vi "FTDI SPI SYS Set.vi"(4 "nCS":u8 max=4 step=1, 5 "ClockRate":u32=50000, 6 "Set Out (0-7)":bool[](array[boolean]), 8 "Use Extra":bool, 10 "Addr":T1 items=["Addr-0", "Addr-1", "Addr-2", "Addr-3", "Addr-4", "Addr-5", "Addr-6", "Addr-7"], 11 "Handler In":u32) -> (0 "error out":errorcluster, 2 "Latch Reg":u32, 3 "Handler Out":u32)   [LabVIEW 2018]
uses:
  PROJEKT/NIKO/Labview/Niko V4/FTDI SPI/Ctl/Sub Addr.ctl
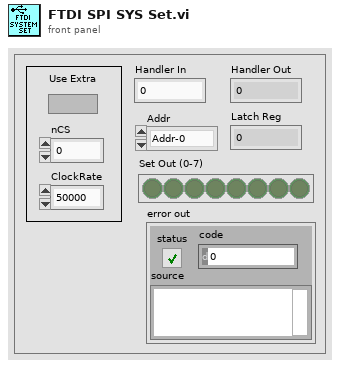
[diagram p1: front panel]
types:
  T1 = typedef "Sub Addr.ctl" = u16
  T2 = cluster{"ClockRate":u32, "LatencyTimer":u8, "configOptions 24-31":i8, "configOptions 16-23":i8, "configOptions 8-15":i8, "configOptions 0-7":u32, "Pin":u32, "reserved":u16}
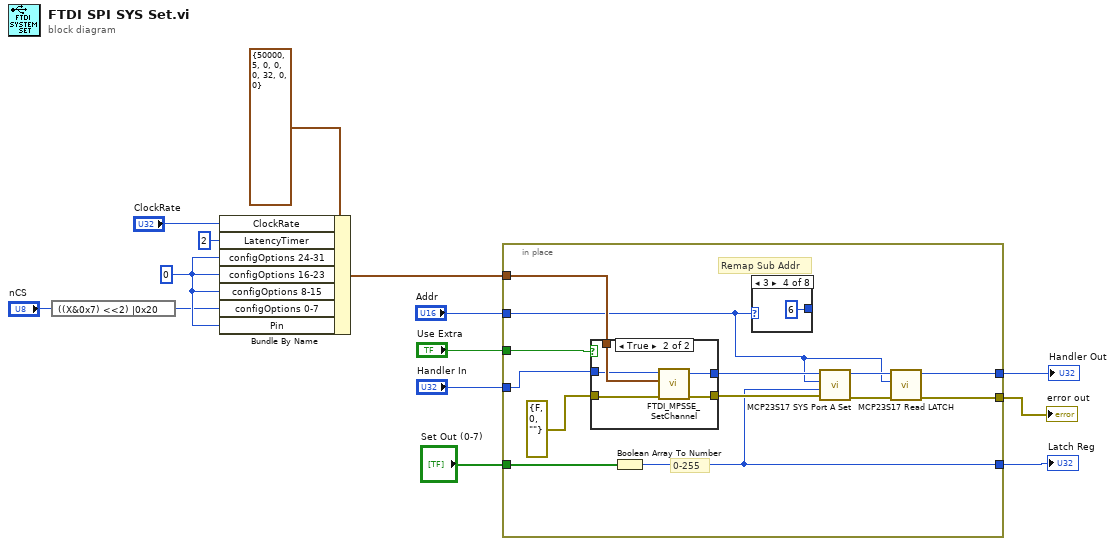
[diagram p0: block diagram]
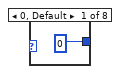
[diagram p2: hidden frame]
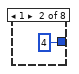
[diagram p3: hidden frame]
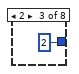
[diagram p4: hidden frame]
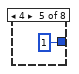
[diagram p5: hidden frame]
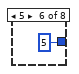
[diagram p6: hidden frame]
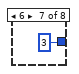
[diagram p7: hidden frame]
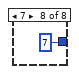
[diagram p8: hidden frame]
diagram:
  w10 = i8 0 ("configOptions 16-23")
  n1 = expression code="((X&0x7) <<2) |0x20"("nCS") -> (w8:u8)
  n2 = Bundle By Name(cluster=T2 {"ClockRate"=50000, "LatencyTimer"=5, "configOptions 24-31"=0, "configOptions 16-23"=0, "configOptions 8-15"=0, "configOptions 0-7"=32, "Pin"=0, "reserved"=0} ("config"), "ClockRate"="ClockRate", "LatencyTimer"=u8 2, "configOptions 24-31"=w10, "configOptions 16-23"=w10, "configOptions 8-15"=w10, "configOptions 0-7"=w8, "Pin"=w10) -> (w6:T2)
  n3 = in-place {
    in-place-border: "Handler In" -> [w27]
    in-place-border: "Addr" -> [w16]
    in-place-border: w6 -> [w25]
    in-place-border: [w17] -> w5
    in-place-border: [w19] -> w4
    in-place-border: "Use Extra" -> [w22]
    in-place-border: "Set Out (0-7)" -> [w21]
    in-place-border: [w15] -> w1
    # "Remap Sub Addr"
    # "0-255"
    n4 = case shown="True" w22 {
      tunnel: w27 -> [w37 w38]
      tunnel: [w37 w41] -> w24
      tunnel: [w36 w42] -> w23
      tunnel: errorcluster {"status"=FALSE, "code"=0, "source"=""} ("error constant") -> [w36 w39]
      tunnel: w25 -> [_ w40]
      frame False {
      }
      frame True {
        n5 = call "FTDI_MPSSE_SetChannel.vi"("error in (no error)"=w39, "config"=w40, "handle"=w38) -> ("error out"=w42:errorcluster, "handle out"=w41:u32)  [unwired: 7 in]
      }
    }
    n6 = Boolean Array To Number(Boolean array=w21) -> (number=w15:u32)
    n7 = case shown="3" w16 {
      tunnel: [0 4 2 6 1 5 3 7] -> _
      frame 0, Default {
      }
      frame 1 {
      }
      frame 2 {
      }
      frame 3 {
      }
      frame 4 {
      }
      frame 5 {
      }
      frame 6 {
      }
      frame 7 {
      }
    }
    n8 = call "MCP23S17 SYS Port A Set.vi"("error in (no error)"=w23, "Channels"=w15, "Addr"=w16, "handle"=w24) -> ("error out"=w20:errorcluster, "handle out"=w18:u32)  [unwired: 6 in]
    n9 = call "MCP23S17 Read LATCH.vi"("error in (no error)"=w20, "Addr"=w16, "handle"=w18) -> ("error out"=w19:errorcluster, "handle out"=w17:u32)  [unwired: 4 in, 3 out]
  }
  "Handler Out" <- w5
  "error out" <- w4
  "Latch Reg" <- w1
